vi "range_of_marks.vi"(9 "lower limit":T1, 10 "upper limit":T1=255, 11 "marksArray":T2[](array[typedef])) -> (3 "Array":T2[](array[typedef]))   [LabVIEW 2015, in "PolyVIEW.lvclass"]
uses:
  PolyVIEW.lvclass
  actors/world/typedefs/markValue_cluster.ctl
  actors/world/typedefs/markValue.ctl
  actors/world/typedefs/markVolume.ctl
  actors/world/world.lvlib
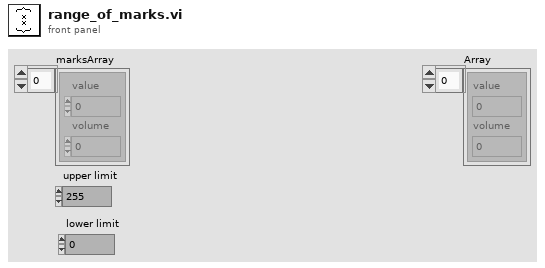
[diagram p1: front panel]
types:
  T1 = typedef "world.lvlib/markValue.ctl" = u8
  T2 = typedef "world.lvlib/markValue_cluster.ctl" = cluster{"value":T1, "volume":T3}
  T3 = typedef "world.lvlib/markVolume.ctl" = u16
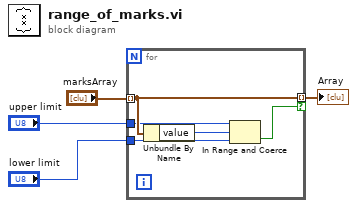
[diagram p0: block diagram]
diagram:
  n1 = for {
    tunnel: "marksArray" -> [w7] mode=indexing
    tunnel: [w7] -> w1 mode=indexing if=w8
    tunnel: "lower limit" -> [w6]
    tunnel: "upper limit" -> [w5]
    n2 = Unbundle By Name(w7) -> ("value"=w9:T1)
    n3 = In Range and Coerce(upper limit=w5, x=w9, lower limit=w6) -> (In Range?=w8:bool)  [unwired: 1 out]
  }
  "Array" <- w1
